vi "ROI2array_inverse_extrinsic.vi"(10 "Pad ROI 1":T1, 11 "Cluster":cluster{"extrinsic":dbl[][], i32[]}) -> (3 "Array":T2(array[cluster]))   [LabVIEW 2017]
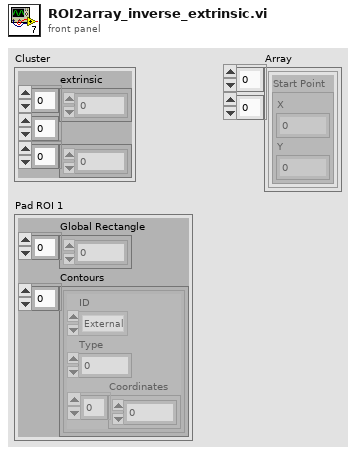
[diagram p1: front panel]
types:
  T1 = cluster{"Global Rectangle":i32[], "Contours":cluster{"ID":enum32{"External", "Internal"}, "Type":u32, "Coordinates":i32[]}[]}
  T2 = cluster{"Start Point":cluster{"X":i32, "Y":i32}}[][]
  T3 = cluster{"Start Point":cluster{"X":i32, "Y":i32}}[]
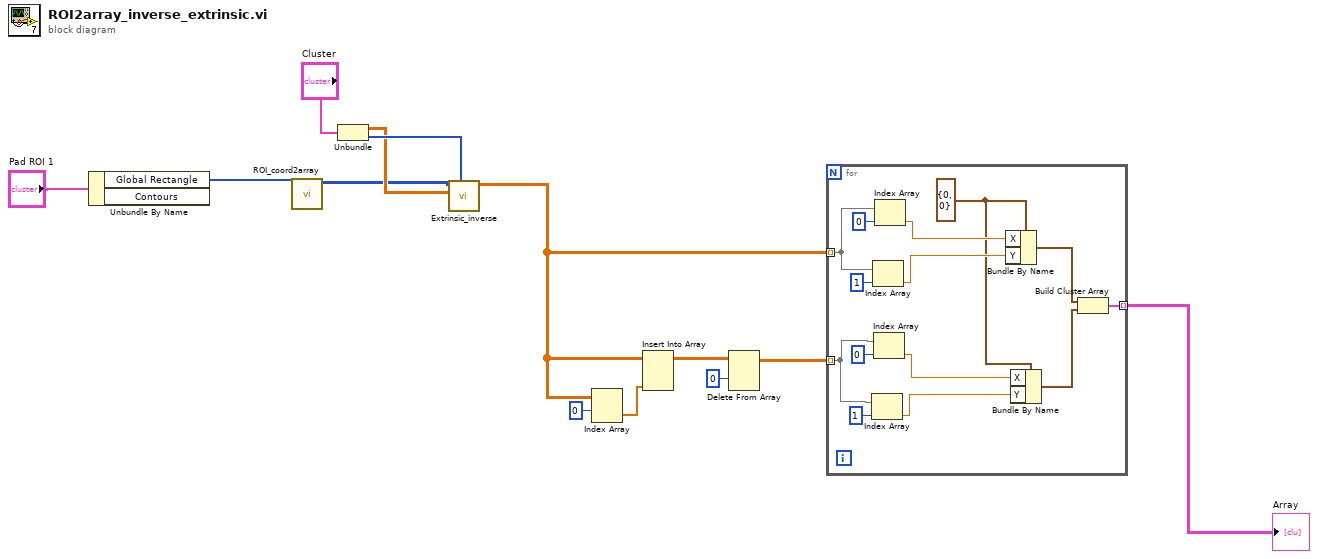
[diagram p0: block diagram]
diagram:
  n1 = Unbundle By Name("Pad ROI 1") -> ("Global Rectangle"=w3:i32[])  [unwired: 1 out]
  n2 = call "ROI_coord2array.vi"("Array in"=w3) -> ("array out"=w11:i32[][])  [unwired: 10 in]
  n3 = Unbundle("Cluster") -> ("extrinsic"=w12:dbl[][], w13:i32[])
  n4 = call "Extrinsic_inverse.vi"("resolution"=w13, "extrinsic"=w12, "X'"=w11) -> ("X'"=w10:dbl[][])  [unwired: 8 in]
  n5 = Index Array(array=w10, index (row)=0 ("index")) -> (element=w5:dbl[])  [unwired: 1 in]
  n6 = Insert Into Array(array=w10, new element=w5) -> (w6:dbl[][])  [unwired: 2 in]
  n7 = Delete From Array(array=w6, index (row)=0 ("length")) -> (array with subset deleted=w8:dbl[][])  [unwired: 2 in, 1 out]
  n8 = for {
    tunnel: w10 -> [w27] mode=indexing
    tunnel: w8 -> [w18] mode=indexing
    tunnel: [w14] -> w9 mode=indexing
    w17 = cluster{"X":i32, "Y":i32} {"X"=0, "Y"=0} ("Start Point")
    n9 = Index Array(array=w18, index=1) -> (element=w22:dbl)
    n10 = Index Array(array=w27, index=1) -> (element=w23:dbl)
    n11 = Index Array(array=w18, index=0) -> (element=w21:dbl)
    n12 = Index Array(array=w27, index=0) -> (element=w24:dbl)
    n13 = Bundle By Name(cluster=w17, "X"=w24, "Y"=w23) -> (w16:cluster{"X":i32, "Y":i32})
    n14 = Bundle By Name(cluster=w17, "X"=w21, "Y"=w22) -> (w15:cluster{"X":i32, "Y":i32})
    n15 = Build Cluster Array(w16, w15) -> (w14:T3)
  }
  "Array" <- w9
